vi "Print.vi"(8 "error in (no error)":errorcluster, 11 "Message Double in":refnum<class "Message Boolean Array.lvclass">) -> (0 "error out":errorcluster, 2 "String":string, 3 "Message Double out":refnum<class "Message Boolean Array.lvclass">)   [LabVIEW 2016, in "Stream Mediator.lvlib" / "Message Boolean Array.lvclass"]
doc: "--\nCopyright © 2017 Composed SystemsI All rights reserved.\n\nAuthor: Jon McBee <jon.mcbee@composed.io>\n\nThis library is provided \"AS IS\" ,WITHOUT WARRANTIES OR\nCONDITIONS OF ANY KIND, either express or implied.\n\nComposed Systems -- composed.io\n\nStream 0.0.1.1\nJon McBee - Composed Systems\nCopyright (c) 2017, Composed Systems"
uses:
  <userlib>/Composed Systems/Stream/Mediator/Classes/Message Boolean Array/Message Boolean Array.lvclass
  C:/Program Files (x86)/National Instruments/LabVIEW 2016/user.lib/Composed Systems/Stream/Mediator/Classes/Message Interface/Message Interface.lvclass
  <userlib>/Composed Systems/Stream/Mediator/Classes/Message Boolean Array/Message Boolean Array.lvclass/Message Boolean Array.ctl
  <userlib>/Composed Systems/Stream/Mediator/Classes/Message Interface/Message Interface.lvclass
  <vilib>/addons/_JKI.lib/Serialization/JSON/JKI JSON Serialization.lvlib
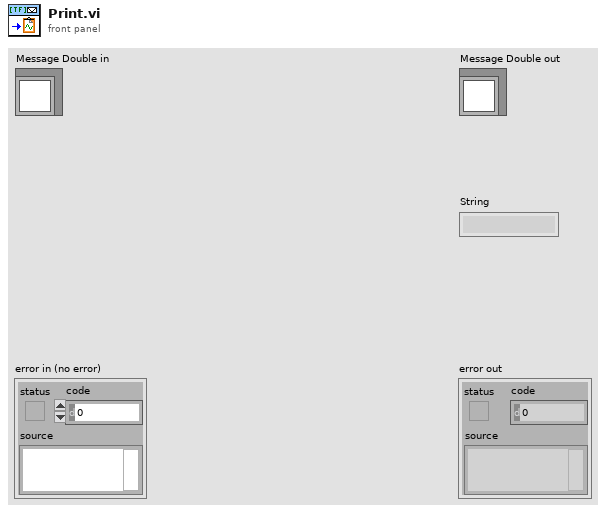
[diagram p1: front panel]
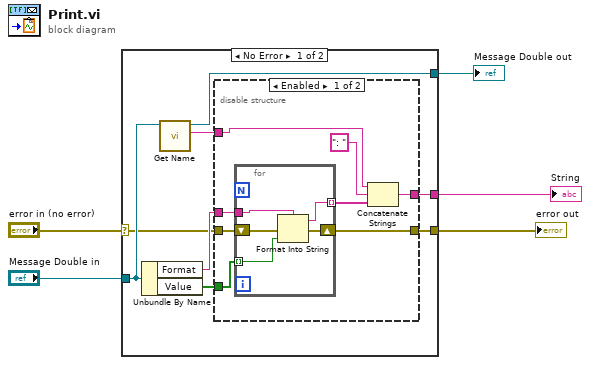
[diagram p0: block diagram]
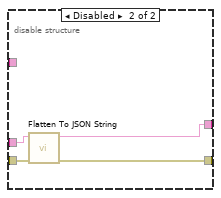
[diagram p2: hidden frame]
diagram:
  n1 = case shown="No Error" "error in (no error)" {
    selector: "error in (no error)" -> [w9 w31]
    tunnel: [w8 w31] -> w4
    tunnel: [w12 w32] -> w2
    tunnel: "Message Double in" -> [w13 w32]
    tunnel: [w6 _] -> w1
    frame No Error {
      n2 = Unbundle By Name(w13) -> ("Format"=w11:string, "Value"=w10:bool[])
      n3 = call <userlib>:"Get Name.vi"("Message Interface in"=w13) -> ("Name"=w7:string, "Message Interface out"=w12:refnum<class "Message Boolean Array.lvclass">)  [unwired: 8 in, 1 out]
      n4 = disable-structure shown="Enabled" {
        disable-tunnel: w11 -> [w21 w30]
        disable-tunnel: w10 -> [w20 _]
        disable-tunnel: w9 -> [w19 w29]
        disable-tunnel: [w18 w28] -> w8
        disable-tunnel: w7 -> [w17 _]
        disable-tunnel: [w14 w27] -> w6
        frame Enabled {
          n5 = for {
            tunnel: w21 -> [w26]
            tunnel: w20 -> [w25] mode=indexing
            shift-right: [w23] -> w18
            shift-left: w19 -> [w24]
            tunnel: [w22] -> w15 mode=indexing
            n6 = Format Into String(format string=w26, error in=w24, w25) -> (resulting string=w22:string, error out=w23:errorcluster)  [unwired: 1 in]
          }
          n7 = Concatenate Strings(w17, ": ", w15) -> (w14:string)
        }
        frame Disabled {
          n8 = call <vilib>:"Flatten To JSON String.vi"("error in (no error)"=w29, "Variant"=w30) -> ("error out"=w28:errorcluster, "JSON String"=w27:string)  [unwired: 8 in]
        }
      }
    }
    frame Error {
    }
  }
  "error out" <- w4
  "Message Double out" <- w2
  "String" <- w1
